vi "LinearFilter_HighPassBW1.vi"(9 "SamplePeriod":dbl format="%13.5p", 11 "TimeConstant":dbl format="%13.5p") -> (3 "LINEAR_FILTER":T1 {"Outputs" format="%13.5g"; "Inputs" format="%13.5g"; "OutputGains" format="%13.5g"; "InputGains" format="%13.5g"})   [LabVIEW 2019, in "Trajectory_Library.lvlib"]
doc: "Creates a 1st order Butterworth high pass filter.\n\nMore information on this type of filter can be found at:\n\n https://en.wikipedia.org/wiki/Butterworth_filter\n\nInputs: \n - timeConstant - The discrete-time time constant in seconds.\n -samplePeriod - The period in seconds between samples taken by the user.\n\nOutputs:\n - Linearfilter - Created datat structure"
uses:
  Trajectory_Library.lvlib
  TypeDef/LINEAR_FILTER.ctl
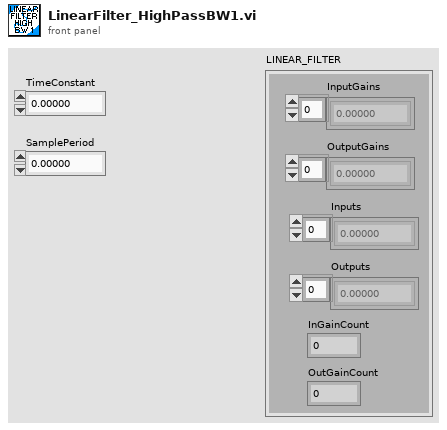
[diagram p1: front panel]
types:
  T1 = typedef "Trajectory_Library.lvlib/LINEAR_FILTER.ctl" = cluster{"InputGains":dbl[], "OutputGains":dbl[], "Inputs":dbl[], "Outputs":dbl[], "InGainCount":i32, "OutGainCount":i32}
  T2 = typedef "WPILib_Math.lvlib/LINEAR_FILTER.ctl" = cluster{"InputGains":dbl[], "OutputGains":dbl[], "Inputs":dbl[], "Outputs":dbl[], "InGainCount":i32, "OutGainCount":i32}
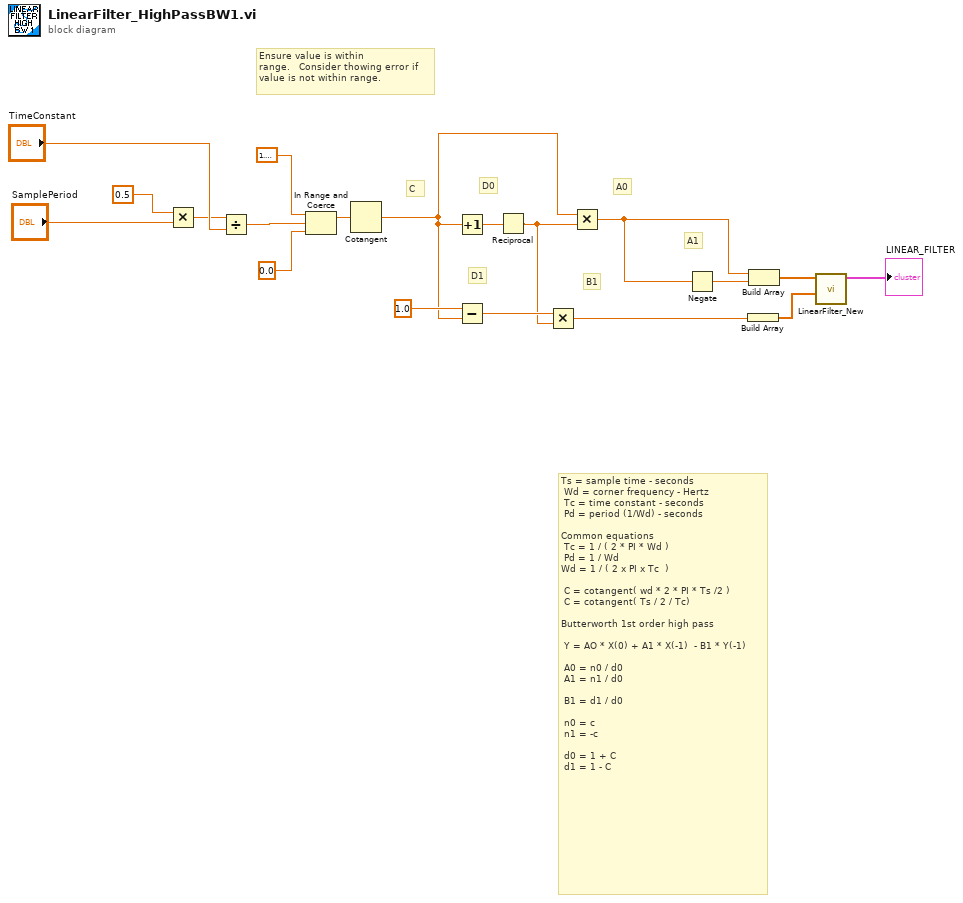
[diagram p0: block diagram]
diagram:
  # "Ensure value is within\nrange.   Consider thowing error if\nvalue is not within range."
  # "B1"
  # "A1"
  # "A0"
  # "Ts = sample time - seconds\n\tWd = corner frequency - Hertz\n\tTc = time constant - seconds\n\tPd = period (1/Wd) - seconds\n\nCommon equations\n\tTc = 1 / ( 2 * PI * Wd )\n\tPd = 1 / Wd\nWd = 1 / ( 2 x PI x Tc  )\n\t\n\tC = cotangent( wd * 2 * PI * Ts /2 )\n C = cotangent( Ts / 2 / Tc)\n\nButterworth 1st order high pass\n\n\tY = AO * X(0) + A1 * X(-1)  - B1 * Y(-1) \n\n\tA0 = n0 / d0\n\tA1 = n1 / d0\n\n\tB1 = d1 / d0\n\n\tn0 = c\n\tn1 = -c\n\n\td0 = 1 + C\n\td1 = 1 - C"
  # "D1"
  # "D0"
  # "C"
  n1 = Multiply(x=0.5, y="SamplePeriod") -> (x*y=w14:dbl)
  n2 = Divide(x=w14, y="TimeConstant") -> (x/y=w6:dbl)
  n3 = In Range and Coerce(upper limit=1.5707963267948966, x=w6, lower limit=0.0) -> (coerced(x)=w5:dbl)  [unwired: 1 out]
  n4 = Cotangent(1:w5) -> (0:w1:dbl)
  n5 = Increment(x=w1) -> (x+1=w4:dbl)
  n6 = Subtract(x=1.0, y=w1) -> (x-y=w10:dbl)
  n7 = Reciprocal(x=w4) -> (1/x=w3:dbl)
  n8 = Multiply(x=w10, y=w3) -> (x*y=w2:dbl)
  n9 = Multiply(x=w1, y=w3) -> (x*y=w9:dbl)
  n10 = Negate(x=w9) -> (-x=w11:dbl)
  n11 = Build Array(w2) -> (w17:dbl[])
  n12 = Build Array(w9, w11) -> (w19:dbl[])
  n13 = call "LinearFilter_New.vi"("OutputGains"=w17, "InputGains"=w19) -> ("LINEAR_FILTER"=→"LINEAR_FILTER":T2)  [unwired: 9 in]
